vi "CreateSerializationSession.vi"(8 "error in":errorcluster) -> (0 "error out":errorcluster, 3 "Serialization Session ID":T1)   [LabVIEW 2019, in "grpc-lvsupport.lvlib"]
uses:
  grpc-lvsupport.lvlib
  grpcId.ctl
  <vilib>/Utility/error.llb/Error Cluster From Error Code.vi
  <resource>/labview_grpc_server.dll
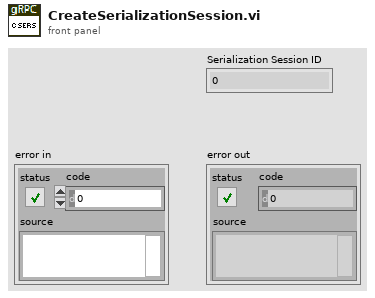
[diagram p1: front panel]
types:
  T1 = typedef "grpc-lvsupport.lvlib/grpcId.ctl" = u64
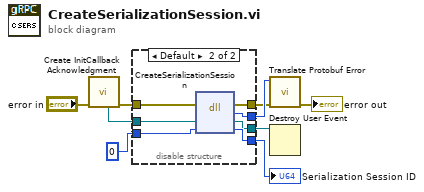
[diagram p0: block diagram]
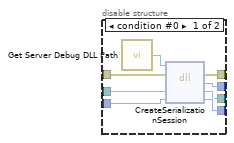
[diagram p2: hidden frame]
diagram:
  n1 = call "Create InitCallback Acknowledgment.vi"("error in (no error)"="error in") -> ("error out"=w4:errorcluster, "Init'd"=w2:refnum<user-event>)  [unwired: 9 in]
  n2 = disable-structure shown="Default" {
    disable-tunnel: [w17 w24] -> w1
    disable-tunnel: u64 0 ("gRPCId") -> [w15 w23]
    disable-tunnel: [w14 w22] -> w7
    disable-tunnel: [w13 w21] -> w5
    disable-tunnel: w4 -> [w12 w20]
    disable-tunnel: [w11 w19] -> w3
    disable-tunnel: w2 -> [w10 w18]
    frame condition #0 {
      n3 = call "Get Server Debug DLL Path.vi"() -> ("DLL Path"=w16:path)
      n4 = dll-call lib="?" fn="CreateSerializationSession"(path in=w16, error in=w12, "InitCallbackAck"=w10, "serializationId"=w15) -> (error out=w17:errorcluster, "return type"=w13:i32, "InitCallbackAck"=w11:refnum<user-event>, "serializationId"=w14:u64)  [unwired: 1 in, 1 out]
    }
    frame condition #1 (active) {
      n5 = dll-call lib="C:/Program Files (x86)/National Instruments/LabVIEW 2024/resource/labview_grpc_server.*" fn="CreateSerializationSession"(error in=w20, "InitCallbackAck"=w18, "serializationId"=w23) -> (error out=w24:errorcluster, "return type"=w21:i32, "InitCallbackAck"=w19:refnum<user-event>, "serializationId"=w22:u64)  [unwired: 2 in, 1 out]
    }
  }
  "Serialization Session ID" <- w7
  n6 = call "Translate Protobuf Error.vi"("error in"=w1, "Error Code"=w5) -> ("error out"=→"error out":errorcluster)  [unwired: 9 in]
  n7 = Destroy User Event(user event=w3) -> ()  [unwired: 1 in, 1 out]
